vi "Robot Move (Celina + Herun).vi"(7 "Reset":bool, 8 "Y axis value":dbl, 9 "Desired Time":dbl, 10 "Desired Distance (ft)":dbl, 11 "Encoder Distance":dbl) -> (3 "Stop State":bool)   [LabVIEW 2014]
uses:
  Drive States.ctl
  <vilib>/Rock Robotics/WPI/RobotDrive/WPI_RobotDriveGetSetRefNum.vi
  <vilib>/Rock Robotics/WPI/RobotDrive/WPI_RobotDriveArcadeDrive_Standard(NoSaturation).vi
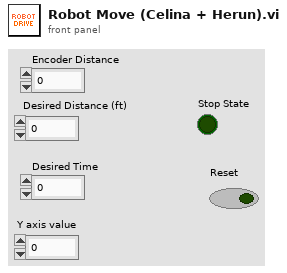
[diagram p1: front panel]
types:
  T1 = typedef "Drive States.ctl" = enum16{"Encoder Reset", "Drive", "Stop"}
  T2 = typedef "WPI_EncoderDevRef.ctl" = cluster{"DevStatus":errorcluster, "EncoderIndex":T3, "CounterIndex":T4, "DistancePerCount":dbl, "Decoding Type":T5}
  T3 = typedef "FPGA_EncoderIdx.ctl" = enum8{"Enc 0", "Enc 1", "Enc 2", "Enc 3", "Enc 4", "Enc 5", "Enc 6", "Enc 7", "Invalid"}
  T4 = typedef "FPGA_CounterCtrSystemIndex.ctl" = enum8{"Ctr 0", "Ctr 1", "Ctr 2", "Ctr 3", "Ctr 4", "Ctr 5", "Ctr 6", "Ctr 7", "Invalid"}
  T5 = typedef "WPI_EncoderType.ctl" = enum16{"1x", "2x", "4x"}
  T6 = typedef "WPI_RobotDriveDevRef.ctl" = cluster{"DevStatus":errorcluster, "Motors[]":T7[], "Square Inputs":bool, "Max Output":dbl}
  T7 = typedef "WPI_MotorControlDeviceRef.ctl" = cluster{"DeviceStatus":errorcluster, "Type":T8, "PWM":cluster{"Controller":T9, "PWM Channel":T10, "DeadBand":T11}, "CAN":cluster{"Device Number":u8, "Control Mode":T12, "Semaphore":T13, "Max Vout":dbl, "TalonSRX Control Mode":T14}, "Invert":bool, "TransformRef":T15, "InvTransformRef":T15}
  T8 = typedef "WPI_MotorControlType.ctl" = enum16{"PWM", "CAN", "CANTalonSRX"}
  T9 = typedef "FPGA_TypedefDigitalModule.ctl" = enum16{"Controller 1"}
  T10 = typedef "FPGA_DIOPWMChannel.ctl" = enum8{"PWM 0", "PWM 1", "PWM 2", "PWM 3", "PWM 4", "PWM 5", "PWM 6", "PWM 7", "PWM 8", "PWM 9", "PWM MXP 0", "PWM MXP 1", "PWM MXP 2", "PWM MXP 3", "PWM MXP 4", "PWM MXP 5", "PWM MXP 6", "PWM MXP 7", "PWM MXP 8", "PWM MXP 9", "Invalid"}
  T11 = typedef "WPI_PWMDeadband.ctl" = cluster{"Name":string, "maxPositivePwm":i32, "minPositivePwm":i32, "centerPwm":i32, "maxNegativePwm":i32, "minNegativePwm":i32, "angularRange":u16}
  T12 = typedef "WPI_CANJaguar_ControlMode.ctl" = enum8{"Percent VBus", "Current", "Speed", "Position", "Voltage"}
  T13 = typedef "Semaphore RefNum" = refnum<k1>
  T14 = typedef "WPI_CANTalonSRX_APIControlMode.ctl" = enum8{"Percent VBus", "Speed", "Position", "Slave", "Unchanged / Invalid"}
  T15 = typedef "WPI_PWMTransform_ConPane.ctl" = refnum<vi>
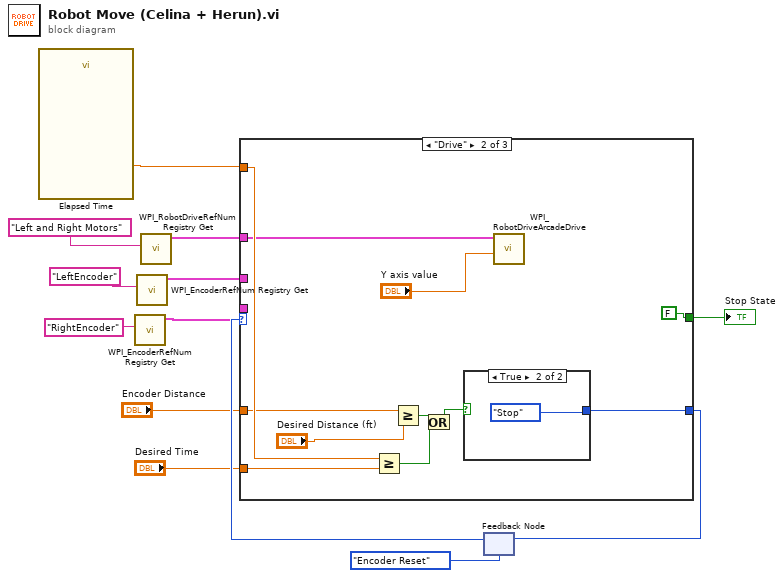
[diagram p0: block diagram]
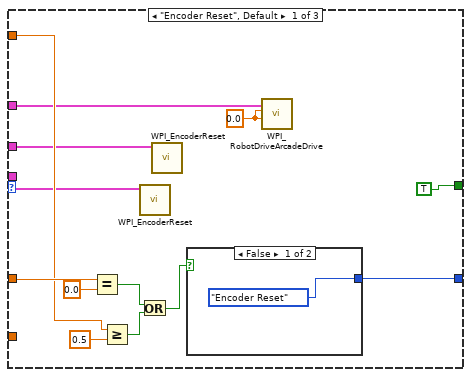
[diagram p2: hidden frame]
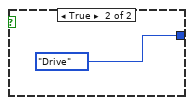
[diagram p3: hidden frame]
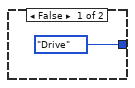
[diagram p4: hidden frame]
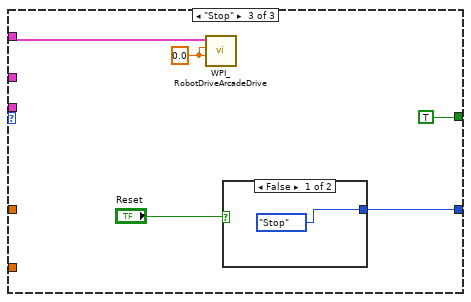
[diagram p5: hidden frame]
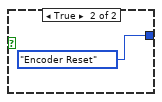
[diagram p6: hidden frame]
diagram:
  n1 = call "Elapsed Time"() -> ("Elapsed Time (s)"=w10:dbl)  [unwired: 12 in, 7 out]
  n2 = call <vilib>:"WPI_EncoderRefNum Registry Get.vi"("refnum name"="RightEncoder") -> ("EncoderDevRef"=w6:T2)  [unwired: 9 in, 1 out]
  n3 = call <vilib>:"WPI_EncoderRefNum Registry Get.vi"("refnum name"="LeftEncoder") -> ("EncoderDevRef"=w5:T2)  [unwired: 9 in, 1 out]
  n4 = call <vilib>:"WPI_RobotDriveRefNum Registry Get.vi"("refnum name"="Left and Right Motors") -> ("RobotDriveDevRef"=w2:T6)  [unwired: 9 in, 1 out]
  n5 = feedback #1(Drive_States."Encoder Reset") -> (w13:T1)
  n6 = case shown="\"Drive\"" w13 {
    tunnel: [w18 w38 w43] -> w11
    tunnel: w10 -> [w22 w37 _]
    tunnel: "Desired Time" -> [_ w36 _]
    tunnel: [TRUE FALSE TRUE] -> w8
    tunnel: "Encoder Distance" -> [w24 w31 _]
    tunnel: w6 -> [w17 _ _]
    tunnel: w5 -> [w16 _ _]
    tunnel: w2 -> [w15 w30 w42]
    frame "Encoder Reset", Default {
      w14 = 0.0 ("Y axis value")
      n7 = Equal?(x=w24, y=0.0) -> (x = y?=w20:bool)
      n8 = Greater Or Equal?(x=w22, y=0.5) -> (x >= y?=w21:bool)
      n9 = call <vilib>:"WPI_EncoderReset.vi"("EncoderDevRef"=w17) -> ()  [unwired: 9 in, 2 out]
      n10 = Or(x=w20, y=w21) -> (x .or. y?=w19:bool)
      n11 = call <vilib>:"WPI_EncoderReset.vi"("EncoderDevRef"=w16) -> ()  [unwired: 9 in, 2 out]
      n12 = case shown="False" w19 {
        tunnel: [Drive_States."Encoder Reset" Drive_States."Drive"] -> w18
        frame False {
        }
        frame True {
        }
      }
      n13 = call-poly <vilib>:"WPI_RobotDriveArcadeDrive.vi"("Y axis value"=w14, "X axis value"=w14, "RobotDriveDevRef"=w15) -> ()  [unwired: 6 in, 3 out]
    }
    frame "Drive" {
      n14 = Greater Or Equal?(x=w37, y=w36) -> (x >= y?=w34:bool)
      n15 = Greater Or Equal?(x=w31, y="Desired Distance (ft)") -> (x >= y?=w35:bool)
      n16 = Or(x=w35, y=w34) -> (x .or. y?=w33:bool)
      n17 = case shown="True" w33 {
        tunnel: [Drive_States."Drive" Drive_States."Stop"] -> w38
        frame False {
        }
        frame True {
        }
      }
      n18 = call-poly <vilib>:"WPI_RobotDriveArcadeDrive.vi"("Y axis value"="Y axis value", "RobotDriveDevRef"=w30) -> ()  [unwired: 7 in, 3 out]
    }
    frame "Stop" {
      w45 = 0.0 ("Y axis value")
      n19 = call-poly <vilib>:"WPI_RobotDriveArcadeDrive.vi"("Y axis value"=w45, "X axis value"=w45, "RobotDriveDevRef"=w42) -> ()  [unwired: 6 in, 3 out]
      n20 = case shown="False" "Reset" {
        tunnel: [Drive_States."Stop" Drive_States."Encoder Reset"] -> w43
        frame False {
        }
        frame True {
        }
      }
    }
  }
  "Stop State" <- w8
  n21 = feedback-in #1(w11) -> ()
